vi "Save Variable Config.vi"(8 "error in (no error)":errorcluster, 10 "Variables":T1, 11 "Path":path) -> (0 "error out":errorcluster)   [LabVIEW 2018, in "File IO.lvlib"]
uses:
  File IO.lvlib
  Public Controls/Variables.ctl
  <vilib>/Utility/NIReport.llb/Report Type.ctl
  <vilib>/Utility/NIReport.llb/NI_report.lvclass
  <vilib>/addons/_office/NI_ReportGenerationToolkit.lvlib
  <vilib>/Utility/NIReport.llb/NI_ReportGenerationCore.lvlib
  <vilib>/Utility/NIReport.llb/Excel/NI_Excel.lvclass
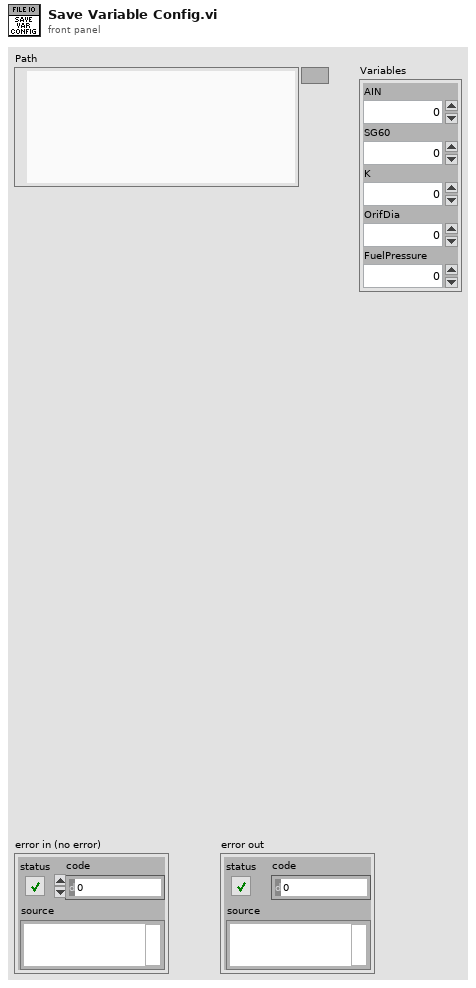
[diagram p1: front panel]
types:
  T1 = typedef "File IO.lvlib/Variables.ctl" = cluster{"AIN":dbl, "SG60":dbl, "K":dbl, "OrifDia":dbl, "FuelPressure":dbl}
  T2 = typedef "NI_ReportGenerationCore.lvlib/Report Type.ctl" = enum16{"HTML", "Word", "Excel"}
  T3 = enum16{"maximized", "minimized", "normal", "no change"}
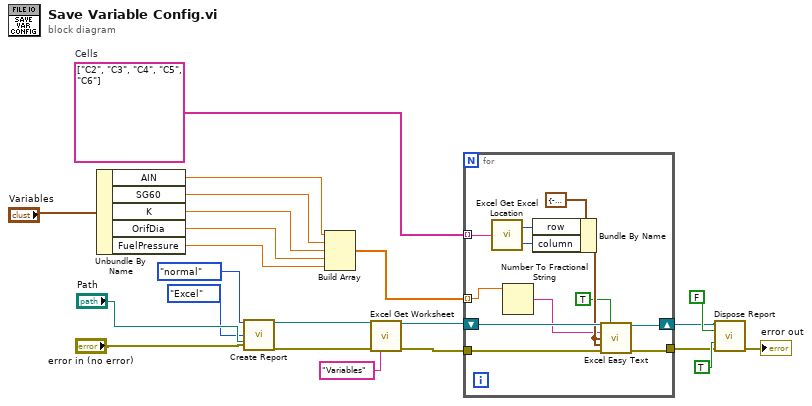
[diagram p0: block diagram]
diagram:
  w19 = string[] ["C2", "C3", "C4", "C5", "C6"]  # Cells
  n1 = Unbundle By Name("Variables") -> ("AIN"=w15:dbl, "SG60"=w16:dbl, "K"=w17:dbl, "OrifDia"=w2:dbl, "FuelPressure"=w1:dbl)
  n2 = call <vilib>:"Create Report.vi"("window state (normal)"=T3."normal", "report type"=Report_Type."Excel", "template (empty)"="Path", "error in (no error)"="error in (no error)") -> ("report out"=w6:refnum<class "NI_report.lvclass">, "error out"=w7:errorcluster)  [unwired: 10 in]
  n3 = Build Array(w15, w16, w17, w2, w1) -> (w18:dbl[])
  n4 = call <vilib>:"Excel Get Worksheet.vi"("report in"=w6, "error in (no error)"=w7, "name (\"\")"="Variables" ("name (\"\")")) -> ("report out"=w12:refnum<class "NI_report.lvclass">, "error out"=w13:errorcluster)  [unwired: 11 in]
  n5 = for {
    shift-right: [w31] -> w8
    shift-left: w12 -> [w32]
    tunnel: [w33] -> w9
    tunnel: w13 -> [w34]
    tunnel: w18 -> [w25] mode=indexing
    tunnel: w19 -> [w26] mode=indexing
    n6 = call <vilib>:"Excel Get Excel Location.vi"("cell's name"=w26) -> ("row"=w28:i32, "column"=w27:i32)
    n7 = Number To Fractional String(number=w25) -> (F-format string=w24:string)  [unwired: 3 in]
    n8 = Bundle By Name(cluster=cluster{"row":i32, "column":i32} {"row"=-1, "column"=-1} ("start (-1, -1)"), "row"=w28, "column"=w27) -> (w29:cluster{"row":i32, "column":i32})
    n9 = call <vilib>:"Excel Easy Text.vi"("report in"=w32, "border? (F)"=TRUE, "text"=w24, "start (-1, -1)"=w29, "end (-1, -1)"=w29, "error in (no error)"=w34) -> ("report out"=w31:refnum<class "NI_report.lvclass">, "error out"=w33:errorcluster)  [unwired: 5 in, 3 out]
  }
  n10 = call-dynamic "Dispose Report.vi"("report in"=w8, "wait until printing completed? (T)"=FALSE, "save changes? (F)"=TRUE, "error in (no error)"=w9) -> ("error out"=→"error out":errorcluster)  [unwired: 11 in]
